vi "Place New Shield.vi"(0 "Shield in":refnum<class "Shield.lvclass">, 1 "Snake":refnum<class "Snake.lvclass">, 2 "Fruit in":refnum<class "Fruit.lvclass">, 3 "Bomb":refnum<class "Bomb.lvclass">[](array[class]), 4 "B Game Size":u16, 5 "error in (no error)":errorcluster) -> (14 "Shield out":refnum<class "Shield.lvclass">, 19 "error out":errorcluster)   [LabVIEW 2021, in "Shield.lvclass"]
uses:
  Shield.lvclass
  C:/Users/poche/Programs/LabVIEW/imposible snake/GameEl_class/GameEl.lvclass
  Fruit_class/Fruit.lvclass
  Snake_class/Snake.lvclass
  Bomb/Bomb.lvclass
  Shield.lvclass/Shield.ctl
  GameEl_class/GameEl.lvclass/GameEl.ctl
  GameEl_class/Read position.vi
  GameEl_class/GameEl.lvclass
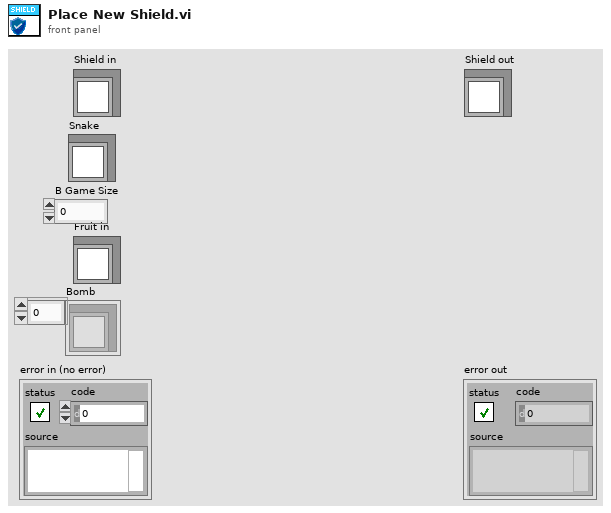
[diagram p1: front panel]
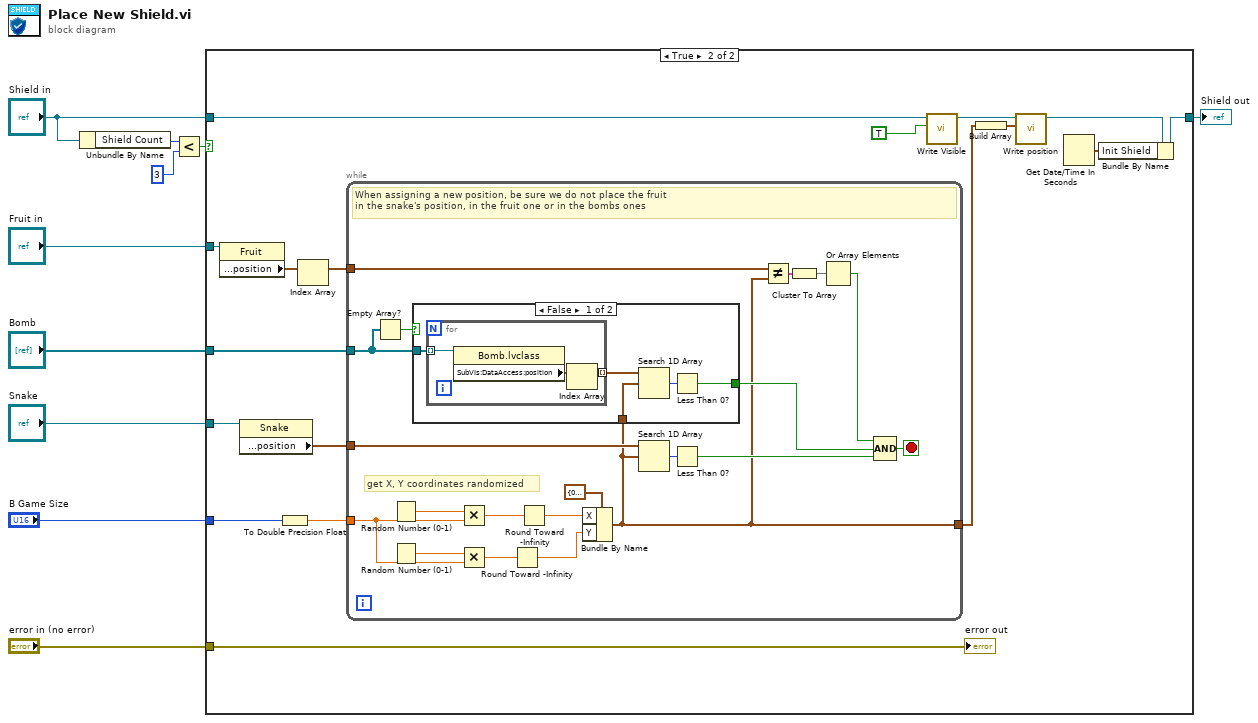
[diagram p0: block diagram]
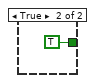
[diagram p3: hidden frame]
diagram:
  n1 = Unbundle By Name("Shield in") -> ("Shield Count"=w3:u8)
  n2 = Less?(x=w3, y=u8 3) -> (x < y?=w1:bool)
  n3 = case shown="True" w1 {
    tunnel: "error in (no error)" -> [_ w28]
    tunnel: "Shield in" -> [w11 w27]
    tunnel: [w11 w26] -> w9
    tunnel: "B Game Size" -> [_ w24]
    tunnel: "Snake" -> [_ w22]
    tunnel: "Bomb" -> [_ w20]
    tunnel: "Fruit in" -> [_ w19]
    frame False {
    }
    frame True {
      n4 = property class="Fruit"(reference=w19) -> ("SubVIs:DataAccess:position"=w18:cluster{"x":dbl, "y":dbl}[])  [unwired: 1 in, 2 out]
      n5 = property class="Snake"(reference=w22) -> ("SubVIs:DataAccess:position"=w21:cluster{"x":dbl, "y":dbl}[])  [unwired: 1 in, 2 out]
      n6 = To Double Precision Float(number=w24) -> (double precision float=w23:dbl)
      n7 = Index Array(array=w18) -> (element=w12:cluster{"x":dbl, "y":dbl})  [unwired: 1 in]
      n8 = while {
        tunnel: w23 -> [w46]
        tunnel: w21 -> [w39]
        tunnel: [w32] -> w15
        tunnel: w20 -> [w35]
        tunnel: w12 -> [w33]
        stop <- w38 stop-if-true
        # "get X, Y coordinates randomized"
        # "When assigning a new position, be sure we do not place the fruit \nin the snake's position, in the fruit one or in the bombs ones"
        n9 = Empty Array?(array=w35) -> (empty?=w34:bool)
        n10 = Random Number (0-1)() -> (number: 0 to 1=w48:dbl)
        n11 = Random Number (0-1)() -> (number: 0 to 1=w47:dbl)
        n12 = Multiply(x=w48, y=w46) -> (x*y=w44:dbl)
        n13 = Multiply(x=w47, y=w46) -> (x*y=w43:dbl)
        n14 = Round Toward -Infinity(1:w43) -> (0:w40:dbl)
        n15 = Round Toward -Infinity(1:w44) -> (0:w41:dbl)
        n16 = Bundle By Name(cluster=cluster{"X":dbl, "Y":dbl} {"X"=0.0, "Y"=0.0} ("Position"), "X"=w41, "Y"=w40) -> (w32:cluster{"X":dbl, "Y":dbl})
        n17 = case shown="False" w34 {
          tunnel: w32 -> [w52 _]
          tunnel: [w50 TRUE] -> w36
          tunnel: w35 -> [w49 _]
          frame False {
            n18 = for {
              tunnel: w49 -> [w56] mode=indexing
              tunnel: [w54] -> w53 mode=indexing
              n19 = property class="Bomb.lvclass"(reference=w56) -> ("SubVIs:DataAccess:position"=w55:cluster{"x":dbl, "y":dbl}[])  [unwired: 1 in, 2 out]
              n20 = Index Array(array=w55) -> (element=w54:cluster{"x":dbl, "y":dbl})  [unwired: 1 in]
            }
            n21 = Search 1D Array(1D array=w53, element=w52) -> (index of element=w51:i32)  [unwired: 1 in]
            n22 = Less Than 0?(x=w51) -> (x < 0?=w50:bool)
          }
          frame True {
          }
        }
        n23 = Search 1D Array(1D array=w39, element=w32) -> (index of element=w42:i32)  [unwired: 1 in]
        n24 = Less Than 0?(x=w42) -> (x < 0?=w37:bool)
        n25 = Not Equal?(x=w33, y=w32) -> (x != y?=w31:cluster{bool, bool})
        n26 = Cluster To Array(cluster=w31) -> (array=w30:bool[])
        n27 = Or Array Elements(Boolean array=w30) -> (logical OR=w29:bool)
        n28 = Compound Arithmetic op=AND(w29, w36, w37) -> (w38:bool)
      }
      n29 = call "Write Visible.vi"("Visible"=TRUE, "GameEl in"=w27) -> ("GameEl out"=w17:refnum<class "Shield.lvclass">)  [unwired: 8 in, 1 out]
      n30 = Build Array(w15) -> (w14:cluster{"X":dbl, "Y":dbl}[])
      n31 = call "Write position.vi"("position"=w14, "GameEl in"=w17) -> ("GameEl out"=w16:refnum<class "Shield.lvclass">)  [unwired: 8 in, 1 out]
      n32 = Get Date/Time In Seconds() -> (seconds since 1Jan1904=w25:timestamp)
      n33 = Bundle By Name(cluster=w16, "Init Shield"=w25) -> (w26:refnum<class "Shield.lvclass">)
      "error out" <- w28
    }
  }
  "Shield out" <- w9
